vi "testGenerateSystemDefinitionReport.vi"(8 "error in (no error)":errorcluster, 11 "TestCase in":refnum<class "VeriStandTestUtilitiesTests.lvclass">) -> (0 "error out":errorcluster, 3 "TestCase out":refnum<class "VeriStandTestUtilitiesTests.lvclass">)   [LabVIEW 2016, in "VeriStandTestUtilitiesTests.lvclass"]
uses:
  VeriStandTestUtilitiesTests.lvclass
  SystemDefinitionInformation.ctl
  TargetInformation.ctl
  ChassisInformation.ctl
  <vilib>/addons/_JKI Toolkits/VI Tester/TestCase.llb/TestCase.lvclass
  VeriStandTestUtilities.lvlib
  C:/Program Files (x86)/National Instruments/LabVIEW 2016/vi.lib/addons/_JKI Toolkits/VI Tester/TestCase.llb/TestCase.lvclass
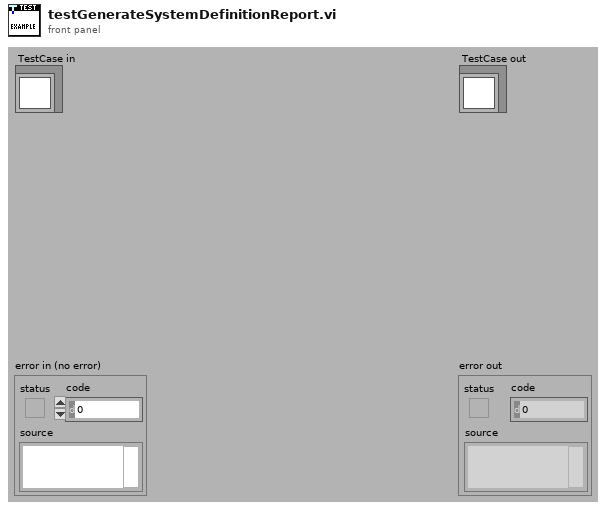
[diagram p1: front panel]
types:
  T1 = typedef "VeriStandTestUtilities.lvlib/SystemDefinitionInformation.ctl" = cluster{"Path":path, "Target Information List":T2[]}
  T2 = typedef "VeriStandTestUtilities.lvlib/TargetInformation.ctl" = cluster{"Name":string, "IP Address":string, "Operating System":string, "Target Rate":dbl, "Chassis List":T3[], "Custom Device List":string[]}
  T3 = typedef "VeriStandTestUtilities.lvlib/ChassisInformation.ctl" = cluster{"Name":string, "Devices":string[]}
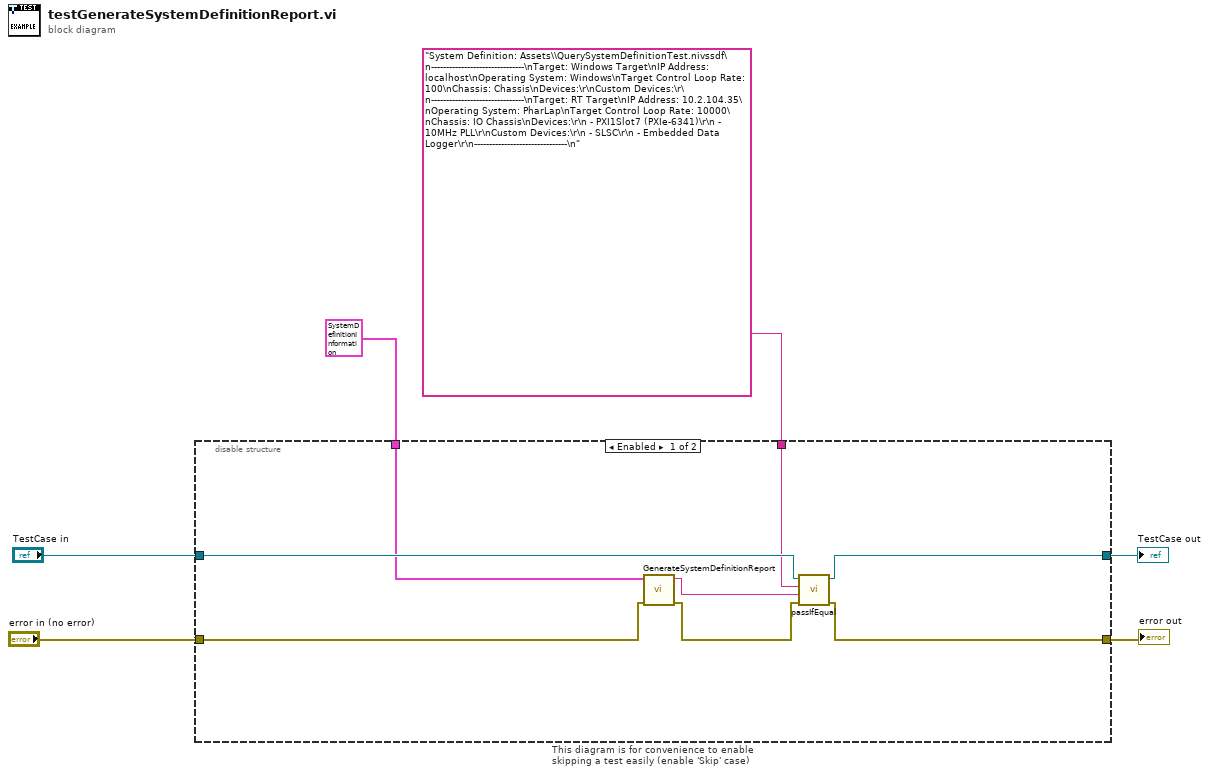
[diagram p0: block diagram]
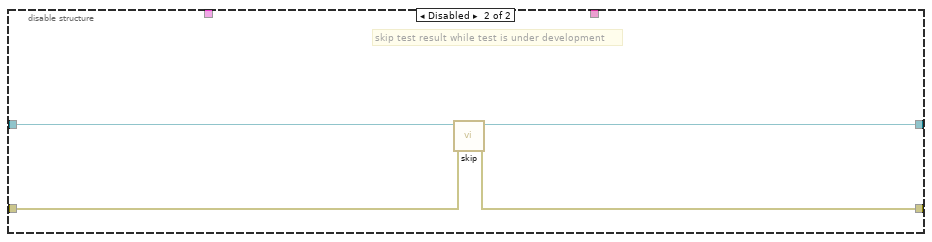
[diagram p2: hidden frame]
diagram:
  n1 = disable-structure "This diagram is for convenience to enable skipping a test easily (enable 'Skip' case)" shown="Enabled" {
    disable-tunnel: "TestCase in" -> [w10 w18]
    disable-tunnel: [w9 w16] -> w3
    disable-tunnel: [w11 w17] -> w5
    disable-tunnel: "error in (no error)" -> [w14 w15]
    disable-tunnel: T1 {"Path"=path "Assets/QuerySystemDefinitionTest.nivssdf", "Target Information List"=[{"Name"="Windows Target", "IP Address"="localhost", "Operating System"="Windows", "Target Rate"=100.0, "Chassis List"=[{"Name"="Chassis", "Devices"=[]}], "Custom Device List"=[]}, {"Name"="RT Target", "IP Address"="10.2.104.35", "Operating System"="PharLap", "Target Rate"=10000.0, "Chassis List"=[{"Name"="IO Chassis", "Devices"=["PXI1Slot7 (PXIe-6341)", "10MHz PLL"]}], "Custom Device List"=["SLSC", "Embedded Data Logger"]}]} ("System Definition Information out") -> [w8 _]
    disable-tunnel: "System Definition: Assets\\QuerySystemDefinitionTest.nivssdf\n-------------------------------\nTarget: Windows Target\nIP Address: localhost\nOperating System: Windows\nTarget Control Loop Rate: 100\nChassis: Chassis\nDevices:\r\nCustom Devices:\r\n-------------------------------\nTarget: RT Target\nIP Address: 10.2.104.35\nOperating System: PharLap\nTarget Control Loop Rate: 10000\nChassis: IO Chassis\nDevices:\r\n - PXI1Slot7 (PXIe-6341)\r\n - 10MHz PLL\r\nCustom Devices:\r\n - SLSC\r\n - Embedded Data Logger\r\n-------------------------------\n" ("Target Information String") -> [w7 _]
    frame Enabled {
      n2 = call "GenerateSystemDefinitionReport.vi"("error in (no error)"=w14, "System Definition Information in"=w8) -> ("error out"=w12:errorcluster, "Target Information String"=w13:string)  [unwired: 8 in]
      n3 = call-dynamic "passIfEqual.vi"("error in (no error)"=w12, "y"=w13, "x"=w7, "TestCase in"=w10) -> ("error out"=w11:errorcluster, "TestCase out"=w9:refnum<class "VeriStandTestUtilitiesTests.lvclass">)  [unwired: 6 in]
    }
    frame Disabled {
      # "skip test result while test is under development"
      n4 = call <vilib>:"skip.vi"("error in (no error)"=w15, "TestCase in"=w18) -> ("error out"=w17:errorcluster, "TestCase out"=w16:refnum<class "VeriStandTestUtilitiesTests.lvclass">)  [unwired: 8 in]
    }
  }
  "error out" <- w5
  "TestCase out" <- w3
